vi "Main.vi"() -> ()   [LabVIEW 2024]
doc: "This template is for the Queued Message Handler design pattern.\n\nThe Event Handling Loop generates messages based on user interface actions.\n\nThe Message Handling Loop processes messages generated by the Event Handling Loop, or by other messages. The messages are string values, so new messages can be added easily to the Message Cases case structure in the Message Handling Loop. Each message cluster can also provide an optional value for Message Data, which is a variant that can be converted to whatever message-specific data is required."
uses:
  Torsjonsrigg/support/MotorBoolControlsIndicators.ctl
  Torsjonsrigg/support/MotorStatusIndicators.ctl
  Torsjonsrigg/controls/UI Data.ctl
  Torsjonsrigg/support/MotorSpeedControls.ctl
  Torsjonsrigg/support/MotorBoolControls.ctl
  <vilib>/Modbus/master/Create Master Instance (TCP).vi
  Torsjonsrigg/support/Message Queue/Enqueue Message (Single).vi
  <vilib>/Utility/error.llb/Error Cluster From Error Code.vi
  <vilib>/addons/control/pid/pid.llb/PID (DBL).vi
  <vilib>/ErrorRing/Error Ring.xnode
  <vilib>/Modbus/master/Modbus Master.lvclass
  Torsjonsrigg/support/Message Queue/Message Queue.lvlib
  Torsjonsrigg/support/User Event - Stop/User Event - Stop.lvlib
  <vilib>/addons/control/pid/NI_PID_pid.lvlib
panel:
  out "Mode Set":string
  in  "Index":i32
  out "Waveform 2":cluster{"X":dbl[], "Y":dbl[]}[](graph) caption="Waveform"
  in  "IP Address of PLC":string="192.168.1.36"
  in  "IPAddress of QuantumX":string="192.168.1.60"
  out "Setpoint Speed 2":dbl format="%.2f"
  out "?":cluster{"X":dbl[], "Y":dbl[]}[](graph)
  out "?":cluster{"X":dbl[], "Y":dbl[]}[](graph)
  out "Torque 1":dbl
  out "Speed Motor 2":dbl format="%.2f"
  out "Speed Motor1":dbl format="%.2f"
  out "Waveform":cluster{"X":dbl[], "Y":dbl[]}[](graph)
  out "Motor Status Indicators":T1
  out "Motor Bool Control Indicators":T2
  in  "Stop":bool
  in  "Setpoint Torque":dbl
  in  "Mode":string(combo)="Synchronus"
  in  "Setpoint Speed":dbl
  in  "Reset":bool
  in  "Start":bool
  in  "Exit":bool
  out "Status":string
  # "Torsion rig Control & Monitoring"
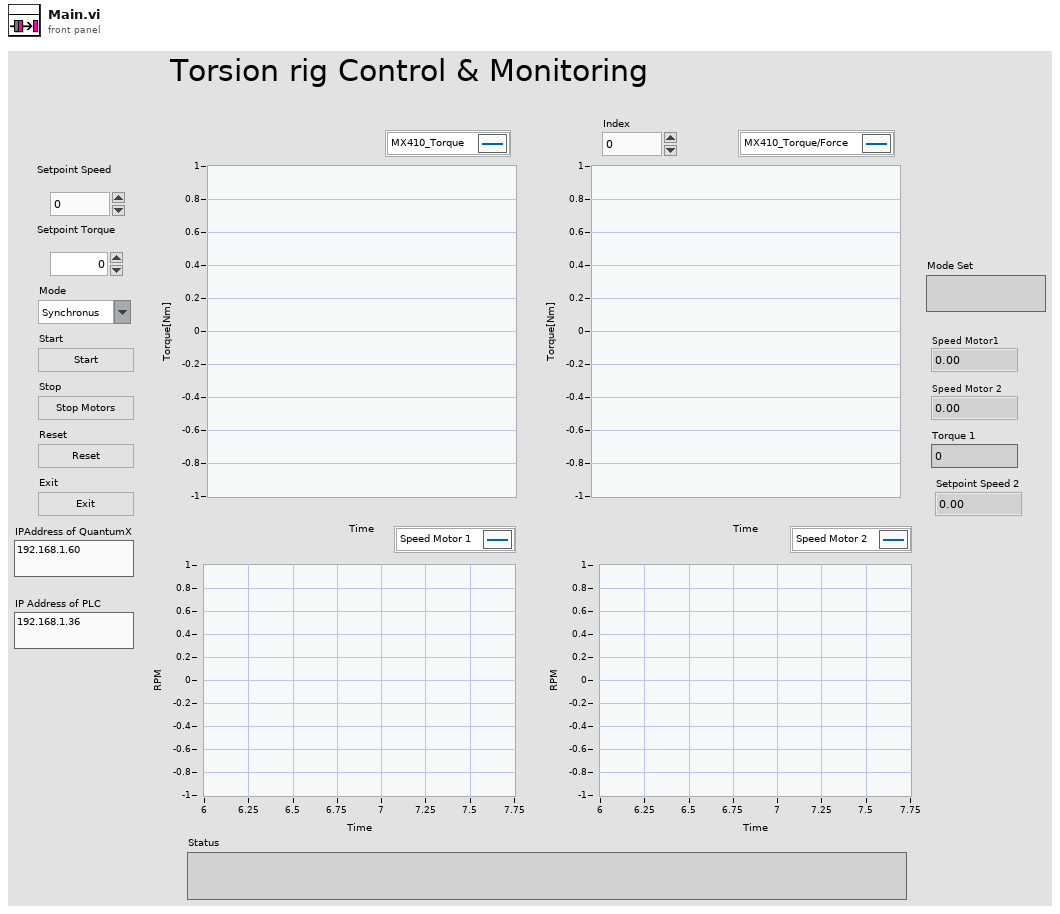
[diagram p1: front panel]
types:
  T1 = typedef "MotorStatusIndicators.ctl" = cluster{"Motor 1 Ok":bool, "Motor 2 ok":bool}
  T2 = typedef "MotorBoolControlsIndicators.ctl" = cluster{"Motors On":bool, "Reset":bool, "Motors Off":bool, "Start Motor 1 ":bool, "Start Motor 2":bool}
  T3 = typedef "MotorBoolControls.ctl" = cluster{"MotorsOn":bool, "Reset":bool, "MotorsOff":bool, "StartMotor1":bool, "StartMotor2":bool}
  T4 = typedef "MotorSpeedControls.ctl" = cluster{"SetSpeed1":dbl, "SetSpeed 2":dbl}
  T5 = typedef "UI Data.ctl" = cluster{"Boolean":bool, "Status":string, "Speed":u32, "Start Ref":refnum<vi>, "Reset":refnum<vi>, "Data Display Ref":refnum<vi>, "Exit Button Ref":refnum<vi>, "Torque":u32, "Async Ref":refnum<vi>, "Sync Ref":string}
  T6 = cluster{"Devices":refnum<k24>[], "Signals":refnum<k24>[]}
  T7 = typedef "Message Queue.lvlib/All Message Queues.ctl" = cluster{"UI":refnum<queue>, "Motor Controller":refnum<queue>, "Logging":refnum<queue>}
  T8 = enum8{"Enabled", "Disabled", "Disabled and Grayed Out"}
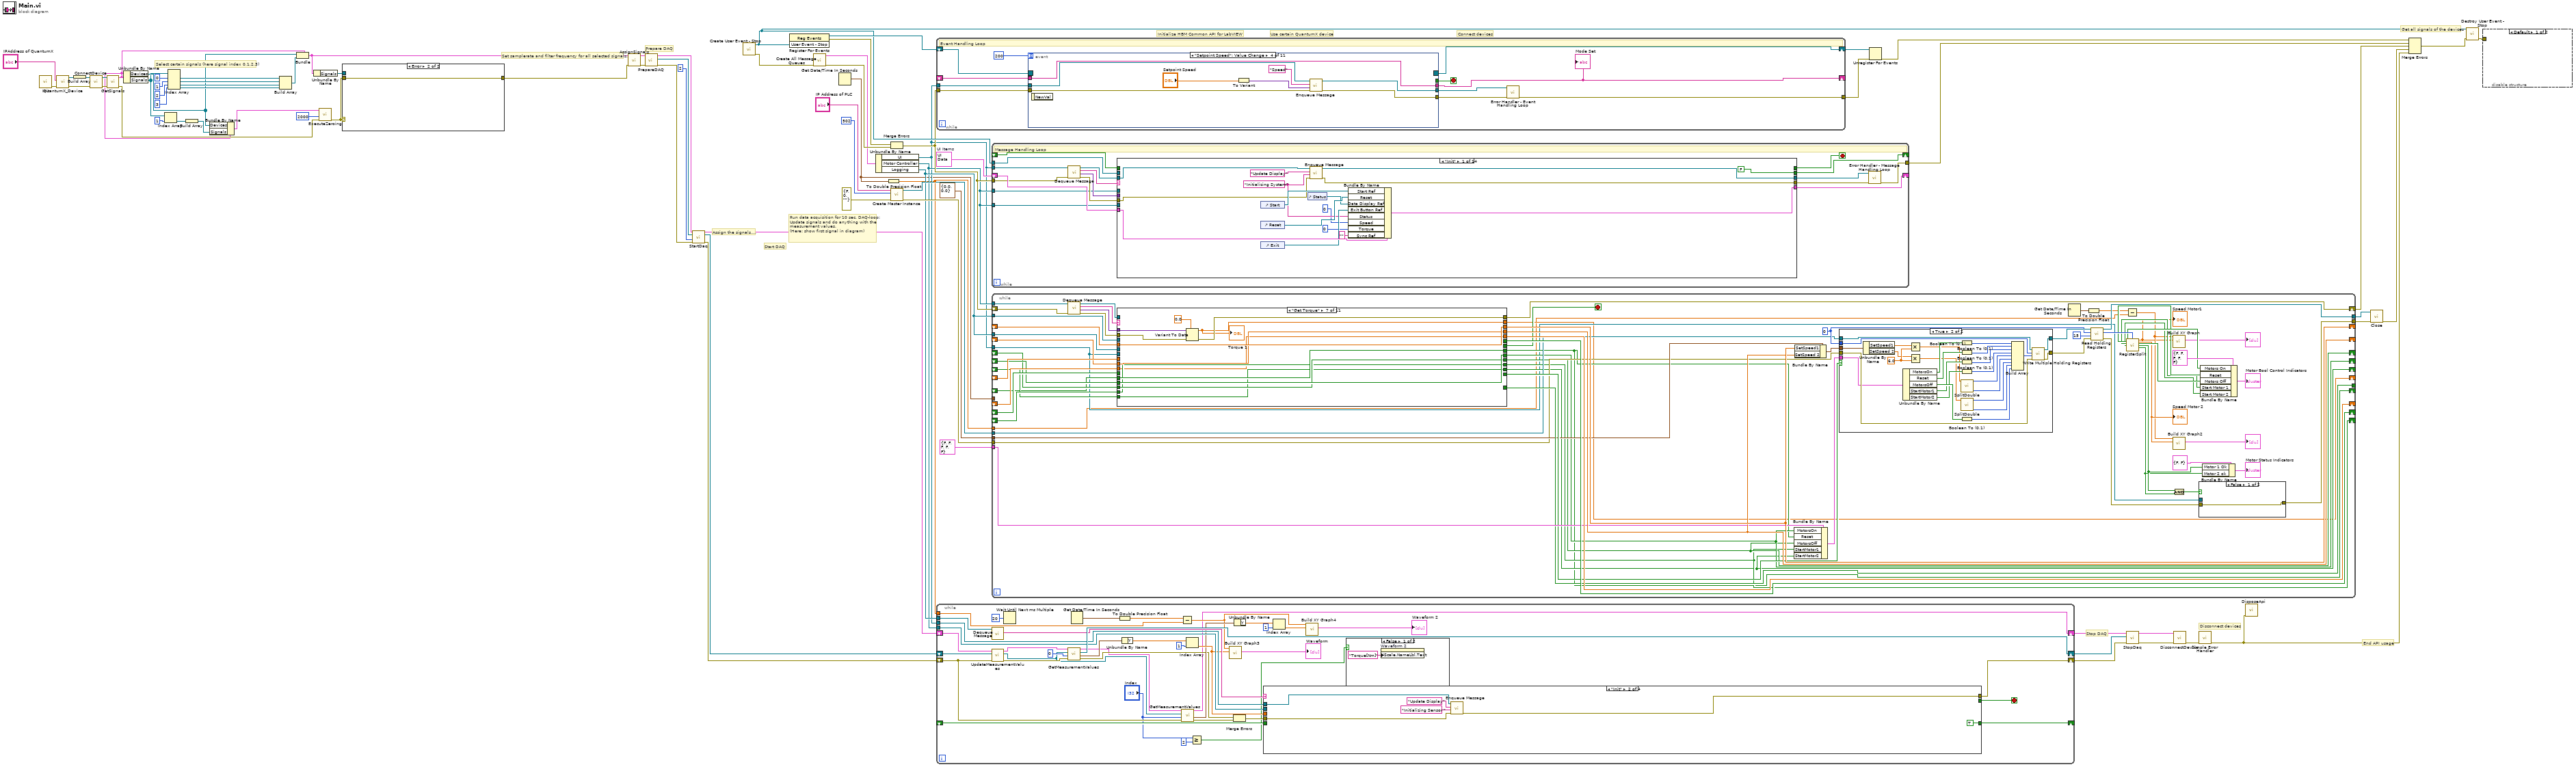
[diagram p0: block diagram]
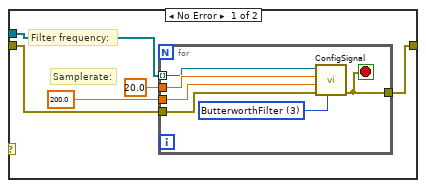
[diagram p2: hidden frame]
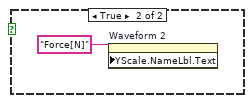
[diagram p3: hidden frame]
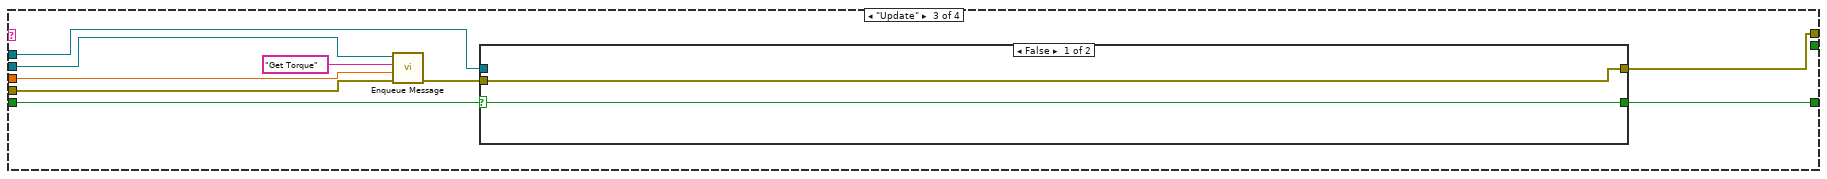
[diagram p5: hidden frame]
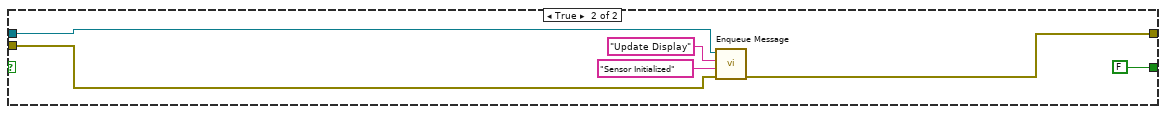
[diagram p6: hidden frame]
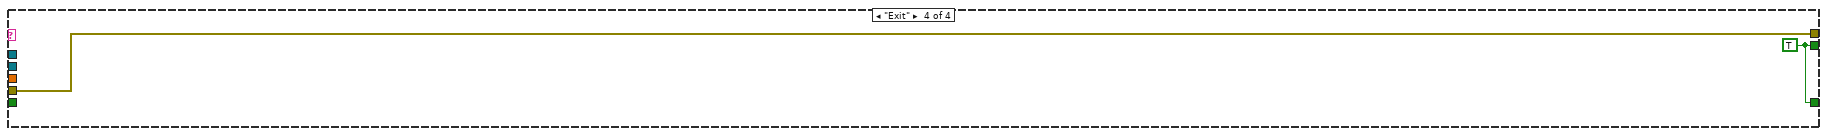
[diagram p7: hidden frame]
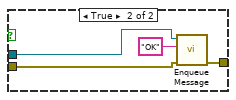
[diagram p8: hidden frame]
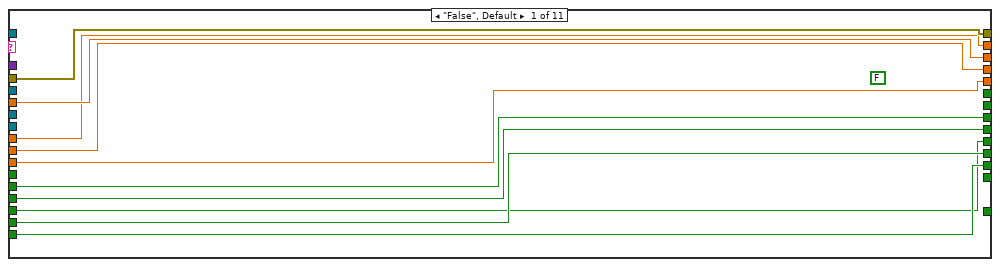
[diagram p10: hidden frame]
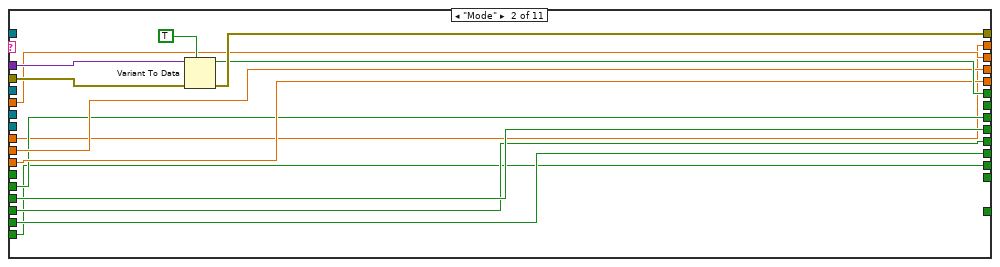
[diagram p11: hidden frame]
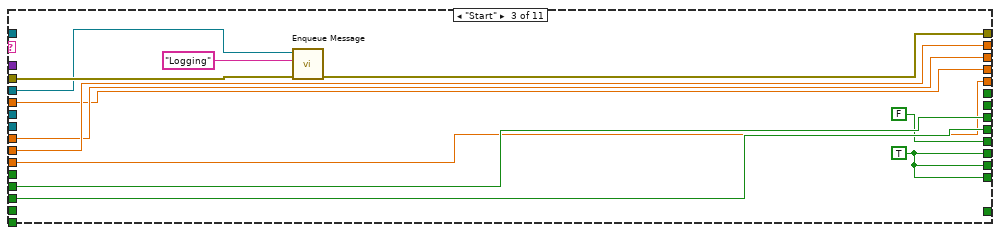
[diagram p12: hidden frame]
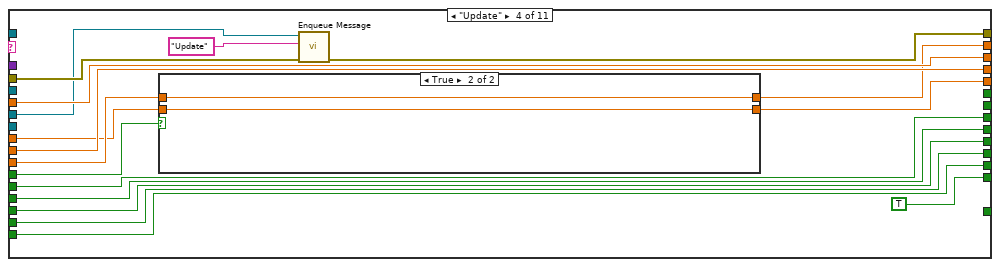
[diagram p13: hidden frame]
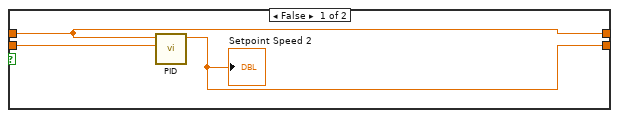
[diagram p14: hidden frame]
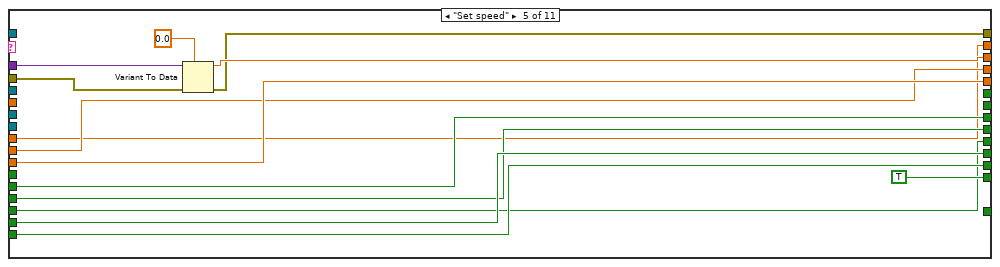
[diagram p15: hidden frame]
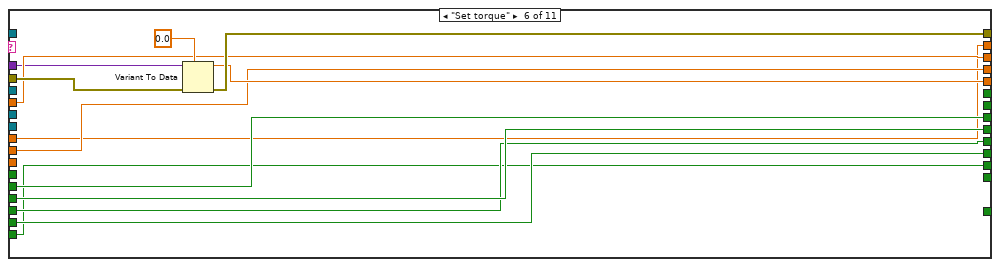
[diagram p16: hidden frame]
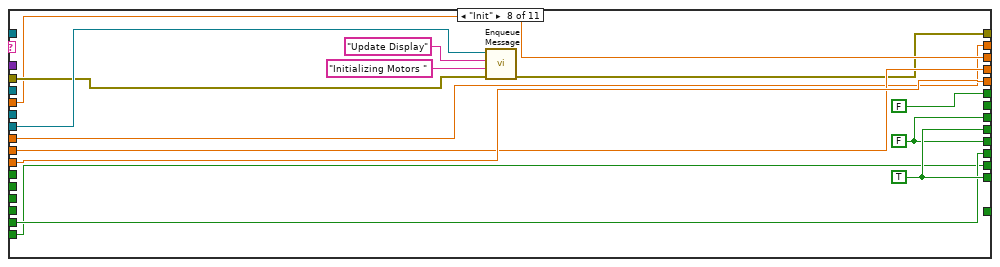
[diagram p17: hidden frame]
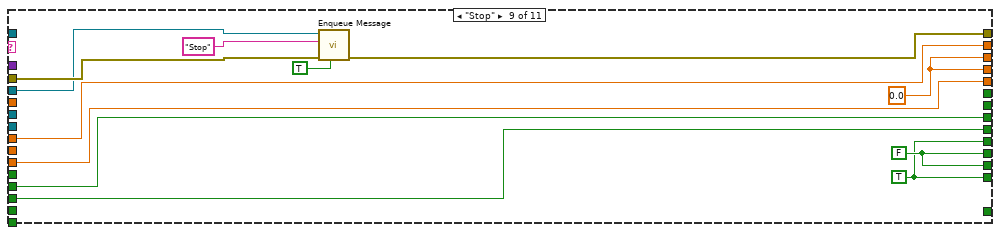
[diagram p18: hidden frame]
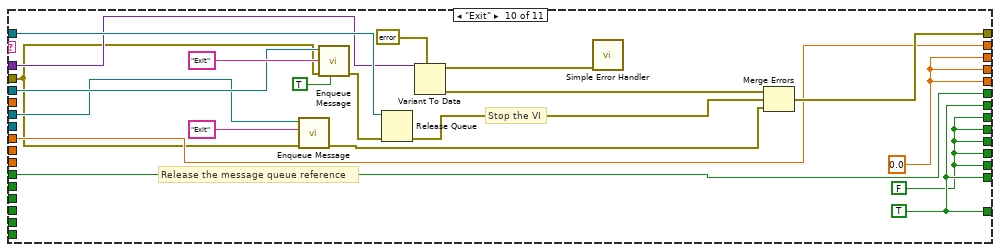
[diagram p19: hidden frame]
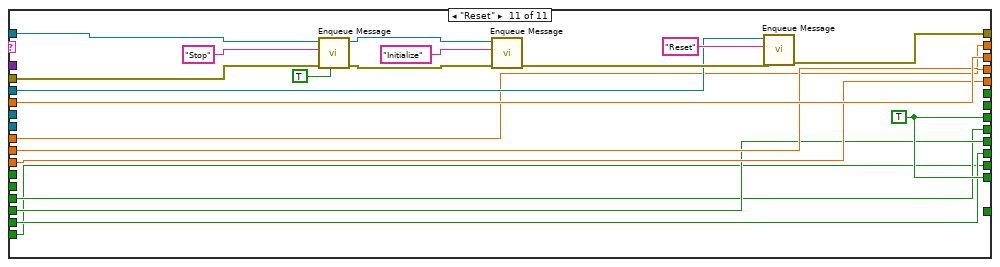
[diagram p20: hidden frame]
diagram:
  w70 = T5 {"Boolean"=FALSE, "Status"="", "Speed"=0, "Start Ref"=refnum, "Reset"=refnum, "Data Display Ref"=refnum, "Exit Button Ref"=refnum, "Torque"=0, "Async Ref"=refnum, "Sync Ref"=""}  # UI Items
  # "Set samplerate and filter frequency for all selected signals."
  # "Run data acquisition for 10 sec. DAQ-loop: Update signals and do anything with the  measurement values.\n(Here: show first signal in diagram)"
  # "Start DAQ"
  # "Prepare DAQ"
  # "Select certain signals (here signal index 0,1,2,3)"
  # "Assign the signals...."
  # "Disconnect devices"
  # "End API usage"
  # "Stop DAQ"
  # "Initialize HBM Common API for LabVIEW"
  # "Get all signals of the devices"
  # "Connect devices"
  # "Use certain QuantumX device"
  n1 = call <userlib>:"Init.vi"() -> ("Error out"=w22:errorcluster)  [unwired: 8 in, 2 out]
  n2 = call <userlib>:"QuantumX_Device.vi"("Error in"=w22, "IPAddress"="IPAddress of QuantumX") -> ("Error out"=w23:errorcluster, "Device"=w20:refnum<k24>)  [unwired: 6 in]
  n3 = Build Array(w20) -> (w19:refnum<k24>[])
  n4 = call <userlib>:"ConnectDevice.vi"("Error in"=w23, "Devices"=w19) -> ("Error out"=w36:errorcluster, "Devices"=w35:refnum<k24>[])  [unwired: 7 in, 1 out]
  n5 = call <userlib>:"GetSignals.vi"("Error in"=w36, "Devices"=w35) -> ("Error out"=w9:errorcluster, "DevicesAndSignals"=w7:T6)  [unwired: 8 in]
  n6 = Unbundle By Name(w7) -> ("Devices"=w11:refnum<k24>[], "Signals"=w10:refnum<k24>[])
  n7 = Index Array(array=w10, index=1) -> (element=w14:refnum<k24>)
  n8 = Index Array(array=w10, index #1=0 ("Index"), index #2=1 ("Index"), index #3=2 ("Index"), index #4=3 ("Index")) -> (element #1=w32:refnum<k24>, element #2=w31:refnum<k24>, element #3=w25:refnum<k24>, element #4=w24:refnum<k24>)
  n9 = Build Array(w14) -> (w15:refnum<k24>[])
  n10 = Bundle By Name(cluster=w7, "Devices"=w11, "Signals"=w15) -> (w6:T6)
  n11 = Build Array(w32, w31, w25, w24) -> (w30:refnum<k24>[])
  n12 = Bundle(cluster=w7, "Devices"=w11, "Signals"=w30) -> (w34:T6)
  n13 = Unbundle By Name(w34) -> ("Signals"=w43:refnum<k24>[])
  n14 = call <userlib>:"ExecuteZeroing.vi"("Error in"=w9, "NumberOfMeasurementValuesToUse"=2000, "DevicesAndSignals"=w6) -> ("Error out"=w8:errorcluster)  [unwired: 7 in, 1 out]
  n15 = case shown="Error" w8 {
    tunnel: w8 -> [w80 w87]
    tunnel: w43 -> [w79 _]
    tunnel: [w78 w87] -> w42
    frame No Error {
      # "Filter frequency:"
      # "Samplerate:"
      n16 = for {
        tunnel: w80 -> [w86]
        tunnel: 200.0 ("SampleRate") -> [w85]
        tunnel: 20.0 ("FilterFrequency") -> [w84]
        tunnel: w79 -> [w83] mode=indexing
        tunnel: [w82] -> w78
        stop <- w82 stop-if-true
        w81 = 3 items=["PresentFilter", "AutoFilter", "BesselFilter", "ButterworthFilter", "HighpassFilter", "LinearPhaseFilter", "NoFilter"] ("FilterType")
        n17 = call <userlib>:"ConfigSignal.vi"("FilterType"=w81, "Error in"=w86, "SampleRate"=w85, "FilterFrequency"=w84, "Signal"=w83) -> ("Error out"=w82:errorcluster)  [unwired: 6 in]
      }
    }
    frame Error {
    }
  }
  n18 = call <userlib>:"AssignSignals.vi"("Error in"=w42, "DevicesAndSignals"=w34) -> ("Error out"=w40:errorcluster, "DevicesAndSignals"=w41:T6)  [unwired: 8 in]
  n19 = call <userlib>:"PrepareDAQ.vi"("Error in"=w40, "DevicesAndSignals"=w41) -> ("Error out"=w37:errorcluster, "DaqMeasurement"=w38:refnum<k24>, "DevicesAndSignals"=w39:T6)  [unwired: 7 in]
  n20 = call <userlib>:"StartDaq.vi"("DevicesAndSignals"=w39, "DaqMeasurement"=w38, "AcquisitionMode"=2, "Error in"=w37) -> ("DevicesAndSignals"=w18:T6, "DaqMeasurement"=w17:refnum<k24>, "Error out"=w16:errorcluster)  [unwired: 7 in, 2 out]
  n21 = call "Create User Event - Stop.vi"() -> ("error out"=w64:errorcluster, "User Event - Stop"=w66:refnum<user-event>)  [unwired: 10 in]
  n22 = register-events(w66) -> (reference out=w67:refnum<event-registration>, error out=w65:errorcluster)  [unwired: 2 in]
  n23 = call "Create All Message Queues.vi"("error in (no error)"=w64) -> ("error out"=w75:errorcluster, "Message Queues out"=w63:T7)  [unwired: 9 in]
  n24 = Get Date/Time In Seconds() -> (seconds since 1Jan1904=w2:timestamp)
  n25 = Unbundle By Name(w63) -> ("UI"=w3:refnum<queue>, "Motor Controller"=w4:refnum<queue>, "Logging"=w5:refnum<queue>)
  n26 = To Double Precision Float(number=w2) -> (double precision float=w1:dbl)
  n27 = Merge Errors(w65, w75) -> (w61:errorcluster)
  n28 = call-poly <vilib>:"Create Master Instance.vi"("error in (no error)"=errorcluster {"status"=FALSE, "code"=0, "source"=""}, "port (502)"=u16 502, "address"="IP Address of PLC") -> ("error out"=w54:errorcluster, "TCP master instance"=w55:refnum<class "Modbus Master.lvclass">)  [unwired: 7 in]
  n29 = while {
    tunnel: w3 -> [w98]
    shift-right: [w96] -> w71
    shift-left: w67 -> [w97]
    tunnel: [w92] -> w68
    tunnel: w61 -> [w91]
    shift-right: [w89] -> _
    shift-left: _ -> [w88]
    stop <- w94 stop-if-true
    # "Event Handling Loop"
    n30 = event shown="[3] \"Setpoint Speed\": Value Change" {
      selector: w97 -> [_ _ _ _ _ _ _ _ _ _ _]
      dyn-events: [_ _ _ _ _ _ _ _ _ _ _] -> w96
      timeout: 200 -> [_ _ _ _ _ _ _ _ _ _ _]
      tunnel: [_ _ _ _ _ _ _ _ "Exit" _ TRUE ("Discard?")] -> w94
      tunnel: w98 -> [w103 w110 w117 w125 w132 w139 w143 w149 w158 w166 w171]
      tunnel: [w100 w108 w114 w122 w129 w138 w142 w146 w157 w165 w168] -> w95
      tunnel: [w102 w109 w116 w124 w131 w137 w143 w148 w156 w164 w171] -> w93
      tunnel: w91 -> [_ w107 w113 w121 w127 w134 w142 w147 w153 w161 w168]
      tunnel: [w99 "Mode" w112 w118 w126 w133 w141 w144 w151 w160 w167] -> w89
      tunnel: w88 -> [w99 _ w112 w118 w126 w133 w141 w144 w151 w160 w167]
      event "Start": Value Change {
        n31 = event-data() -> ()  [unwired: 1 in, 1 out]
        n32 = call-poly "Enqueue Message.vi"("Message"="Start", "Message Queue"=w103) -> ("error out"=w100:errorcluster, "dup Message Queue"=w102:refnum<queue>)  [unwired: 8 in]
      }
      event "Mode": Value Change {
        n33 = event-data() -> ()  [unwired: 1 in, 1 out]
        n34 = property on="Mode" class="CmbBox"("DisabledEnum"=T8."Disabled and Grayed Out" ("Disabled")) -> ()  [unwired: 2 in, 2 out]
        n35 = call-poly "Enqueue Message.vi"("error in (no error)"=w107, "Message Data"="Mode", "Message"="Mode", "Message Queue"=w110) -> ("error out"=w108:errorcluster, "dup Message Queue"=w109:refnum<queue>)  [unwired: 6 in]
      }
      event "Reset": Value Change {
        n36 = event-data() -> ()  [unwired: 1 in, 1 out]
        n37 = call-poly "Enqueue Message.vi"("error in (no error)"=w113, "Message"="Reset", "Message Queue"=w117) -> ("error out"=w114:errorcluster, "dup Message Queue"=w116:refnum<queue>)  [unwired: 7 in]
        n38 = property on="Mode" class="CmbBox"("DisabledEnum"=T8."Enabled" ("Disabled")) -> ()  [unwired: 2 in, 2 out]
      }
      event "Setpoint Speed": Value Change {
        n39 = event-data() -> ()  [unwired: 1 in, 1 out]
        n40 = To Variant(anything="Setpoint Speed") -> (Variant=w119:variant)
        n41 = call-poly "Enqueue Message.vi"("error in (no error)"=w121, "Message Data"=w119, "Message"="Speed", "Message Queue"=w125) -> ("error out"=w122:errorcluster, "dup Message Queue"=w124:refnum<queue>)  [unwired: 6 in]
      }
      event "Setpoint Torque": Value Change {
        n42 = event-data() -> ()  [unwired: 1 in, 1 out]
        n43 = call-poly "Enqueue Message.vi"("error in (no error)"=w127, "Message Data"="Setpoint Torque", "Message"="Torque", "Message Queue"=w132) -> ("error out"=w129:errorcluster, "dup Message Queue"=w131:refnum<queue>)  [unwired: 6 in]
      }
      event Panel Close? {
        n44 = event-data() -> ()  [unwired: 1 in, 1 out]
        n45 = call-poly "Enqueue Message.vi"("Priority Message? (F)"=TRUE, "error in (no error)"=w134, "Message"="Confirm Quit", "Message Queue"=w139) -> ("error out"=w138:errorcluster, "dup Message Queue"=w137:refnum<queue>)  [unwired: 6 in]
        n46 = event-data("Discard?"=TRUE) -> ()  [unwired: 1 in, 1 out]
      }
      event Application Instance Close {
        n47 = event-data() -> ()  [unwired: 1 in, 1 out]
      }
      event Timeout {
        n48 = event-data() -> ()  [unwired: 1 in, 3 out]
        n49 = call-poly "Enqueue Message.vi"("error in (no error)"=w147, "Message"="Update", "Message Queue"=w149) -> ("error out"=w146:errorcluster, "dup Message Queue"=w148:refnum<queue>)  [unwired: 7 in]
      }
      event "Exit": Value Change {
        n50 = event-data() -> ()  [unwired: 1 in, 1 out]
        n51 = call-poly "Enqueue Message.vi"("Priority Message? (F)"=TRUE, "error in (no error)"=w153, "Message"="Exit", "Message Queue"=w158) -> ("error out"=w157:errorcluster, "dup Message Queue"=w156:refnum<queue>)  [unwired: 6 in]
        n52 = property on="Mode" class="CmbBox"("DisabledEnum"=T8."Enabled" ("Disabled")) -> ()  [unwired: 2 in, 2 out]
      }
      event "Stop": Value Change {
        n53 = event-data() -> ()  [unwired: 1 in, 1 out]
        n54 = call-poly "Enqueue Message.vi"("Priority Message? (F)"=TRUE, "error in (no error)"=w161, "Message"="Stop", "Message Queue"=w166) -> ("error out"=w165:errorcluster, "dup Message Queue"=w164:refnum<queue>)  [unwired: 6 in]
        n55 = property on="Mode" class="CmbBox"("DisabledEnum"=T8."Enabled" ("Disabled")) -> ()  [unwired: 2 in, 2 out]
      }
      event User Event {
        n56 = event-data() -> ()  [unwired: 1 in, 1 out]
        n57 = local write "Status"("\"Exit\" button pressed" ("VI Stopped")) -> ()
      }
    }
    "Mode Set" <- w89
    n58 = call "Error Handler - Event Handling Loop.vi"("error in (no error)"=w95, "Message Queue"=w93) -> ("dup error in"=w92:errorcluster)  [unwired: 8 in, 1 out]
  }
  n59 = while {
    shift-right: [w175] -> w45
    shift-left: w18 -> [w209]
    shift-right: [w207] -> w50
    shift-left: w17 -> [w208]
    shift-right: [w199] -> w44
    shift-left: w16 -> [w180]
    tunnel: w5 -> [w210]
    tunnel: w4 -> [w200]
    tunnel: w3 -> [w202]
    shift-right: [w198] -> _
    shift-left: _ -> [w197]
    tunnel: w1 -> [w193]
    stop <- w201 stop-if-true
    n60 = call "Dequeue Message.vi"("Message Queue"=w210) -> ("Message"=w203:string)  [unwired: 7 in, 3 out]
    n61 = call <userlib>:"UpdateMeasurementValues.vi"("Error in"=w180, "DaqMeasurement"=w208, "DevicesAndSignals"=w209) -> ("Error out"=w204:errorcluster, "DaqMeasurement"=w181:refnum<k24>, "DevicesAndSignals"=w188:T6)  [unwired: 6 in]
    n62 = Wait Until Next ms Multiple(millisecond multiple=u32 20 ("Vielfache von ms")) -> ()  [unwired: 1 out]
    n63 = call <userlib>:"GetMeasurementValues.vi"("Error in"=w204, "Index"=0 ("Signal index to display"), "DaqMeasurement"=w181, "DevicesAndSignals"=w188) -> ("Error out"=w179:errorcluster, "Waveform"=w196:waveform(dbl), "DaqMeasurement"=w207:refnum<k24>, "DevicesAndSignals"=w176:T6)  [unwired: 2 in, 2 out]
    n64 = Get Date/Time In Seconds() -> (seconds since 1Jan1904=w195:timestamp)
    n65 = To Double Precision Float(number=w195) -> (double precision float=w194:dbl)
    n66 = Unbundle By Name(w196) -> ("Y"=w192:dbl[])
    n67 = Subtract(x=w194, y=w193) -> (x-y=w183:dbl)
    n68 = call <userlib>:"GetMeasurementValues.vi"("Error in"=w180, "Index"="Index", "DaqMeasurement"=w181, "DevicesAndSignals"=w176) -> ("Error out"=w177:errorcluster, "Waveform"=w184:waveform(dbl), "DevicesAndSignals"=w175:T6)  [unwired: 2 in, 3 out]
    n69 = Index Array(array=w192, index=1) -> (element=w189:dbl)
    n70 = Greater Or Equal?(x="Index", y=2) -> (x >= y?=w172:bool)
    n71 = call "Build XY Graph3"("Y Input"=w189, "X Input"=w183) -> ("XY Graph"=→"Waveform":cluster{"X":dbl[], "Y":dbl[]}[])  [unwired: 8 in, 1 out]
    n72 = Merge Errors(w179, w177) -> (w178:errorcluster)
    n73 = Unbundle By Name(w184) -> ("Y"=w187:dbl[])
    n74 = case shown="\"Init\"" w203 {
      tunnel: w202 -> [_ w220 w222 _]
      tunnel: [_ _ _ w238] -> w201
      tunnel: w178 -> [w214 w217 w229 w239]
      tunnel: w200 -> [_ _ w227 _]
      tunnel: [w214 w216 w224 w239] -> w199
      tunnel: [w213 TRUE w223 w238] -> w198
      tunnel: w197 -> [w213 _ w226 _]
      tunnel: w189 -> [_ _ w221 _]
      frame "False", Default {
      }
      frame "Init" {
        n75 = call-poly "Enqueue Message.vi"("error in (no error)"=w217, "Message Data"="Initializing Sensor ", "Message"="Update Display", "Message Queue"=w220) -> ("error out"=w216:errorcluster)  [unwired: 6 in, 1 out]
      }
      frame "Update" {
        n76 = call-poly "Enqueue Message.vi"("error in (no error)"=w229, "Message Data"=w221, "Message"="Get Torque", "Message Queue"=w227) -> ("error out"=w225:errorcluster)  [unwired: 6 in, 1 out]
        n77 = case shown="False" w226 {
          selector: w226 -> [w230 _]
          tunnel: [w231 w235] -> w224
          tunnel: w225 -> [w231 w234]
          tunnel: [w230 FALSE] -> w223
          tunnel: w222 -> [_ w232]
          frame False {
          }
          frame True {
            n78 = call-poly "Enqueue Message.vi"("error in (no error)"=w234, "Message Data"="Sensor Initialized", "Message"="Update Display", "Message Queue"=w232) -> ("error out"=w235:errorcluster)  [unwired: 6 in, 1 out]
          }
        }
      }
      frame "Exit" {
        w238 = TRUE
      }
    }
    n79 = Index Array(array=w187, index=1) -> (element=w182:dbl)
    n80 = call "Build XY Graph4"("Y Input"=w182, "X Input"=w183) -> ("XY Graph"=→"Waveform 2":cluster{"X":dbl[], "Y":dbl[]}[])  [unwired: 8 in, 1 out]
    n81 = case shown="False" w172 {
      frame False {
        n82 = property on="Waveform 2" class="XYGraph (strict)"("YScale.NameLbl.Text"="Torque[Nm]" ("Y Scale.Name Label.Text")) -> ()  [unwired: 2 in, 2 out]
      }
      frame True {
        n83 = property on="Waveform 2" class="XYGraph (strict)"("YScale.NameLbl.Text"="Force[N]" ("Y Scale.Name Label.Text")) -> ()  [unwired: 2 in, 2 out]
      }
    }
  }
  n84 = while {
    shift-right: [w255] -> _
    shift-left: w70 -> [w256]
    tunnel: w66 -> [w250]
    tunnel: w61 -> [w253]
    tunnel: [w252] -> w74
    tunnel: w3 -> [w248]
    tunnel: w4 -> [w245]
    tunnel: w4 -> [w242]
    shift-right: [w241] -> _
    shift-left: _ -> [w240]
    stop <- w254 stop-if-true
    # "Message Handling Loop"
    n85 = call "Dequeue Message.vi"("error in (no error)"=w253, "Message Queue"=w248) -> ("error out"=w246:errorcluster, "Message Data"=w247:variant, "Message"=w249:string, "dup Message Queue"=w244:refnum<queue>)  [unwired: 6 in]
    n86 = case "Message Cases" shown="\"Init\"" w249 {
      selector: w249 -> [_ w275 _ _ _ _ _ _ _ _ _ _ _ w388]
      tunnel: [w272 w277 w282 _ w290 w304 w316 w327 w337 w351 w357 w367 w382 w389] -> w251
      tunnel: w256 -> [w271 w280 w286 w288 w293 w309 w321 w332 w343 w352 w356 w368 w385 w390]
      tunnel: [w270 w280 w286 w288 w293 w309 w321 w332 w343 w352 w356 w368 w385 w390] -> w255
      tunnel: [_ _ _ _ _ _ _ _ _ _ _ _ TRUE _] -> w254
      tunnel: w250 -> [_ _ _ _ _ _ _ _ _ _ _ _ w381 _]
      tunnel: w247 -> [_ w279 _ _ _ w302 w314 _ _ w347 w355 _ w376 _]
      tunnel: w246 -> [w260 w278 w284 _ w291 _ w313 _ w338 w346 w354 _ w371 _]
      tunnel: w245 -> [_ w276 w285 _ _ w303 w317 w328 w336 _ _ _ w372 _]
      tunnel: w244 -> [w261 w274 _ _ _ w301 w312 w324 w335 w345 _ w363 w377 w387]
      tunnel: [w259 w274 _ _ _ w300 w311 w323 w334 w345 _ w362 _ w387] -> w243
      tunnel: w242 -> [_ _ _ _ w292 _ _ _ _ _ _ _ _ _]
      tunnel: [FALSE w273 w281 TRUE w289 w299 w310 w322 w333 w344 w353 FALSE w369 w386] -> w241
      tunnel: w240 -> [_ w273 w281 _ w289 w299 w310 w322 w333 w344 w353 _ w369 w386]
      frame "Init" {
        w264 = "Initializing System" ("Initial Message")
        # "Initialize - All initialization work should take place in this message, since other loops can potentially enqueue messages that execute immediately after this one."
        n87 = control-ref of="Start"() -> (w269:refnum<vi>)
        n88 = control-ref of="Reset"() -> (w268:refnum<vi>)
        n89 = control-ref of="Exit"() -> (w266:refnum<vi>)
        n90 = control-ref of="Status"() -> (w267:refnum<vi>)
        n91 = call-poly "Enqueue Message.vi"("error in (no error)"=w260, "Message Data"=w264, "Message"="Update Display", "Message Queue"=w261) -> ("error out"=w272:errorcluster, "dup Message Queue"=w259:refnum<queue>)  [unwired: 6 in]
        n92 = Bundle By Name(cluster=w271, "Start Ref"=w269, "Reset"=w268, "Data Display Ref"=w267, "Exit Button Ref"=w266, "Status"=w264, "Speed"=u32 0, "Torque"=u32 0, "Sync Ref"="") -> (w270:T5)
      }
      frame "Mode" {
        # "Something - Replace this message with functionality for your own application."
        n93 = call-poly "Enqueue Message.vi"("error in (no error)"=w278, "Message Data"=w279, "Message"=w275, "Message Queue"=w276) -> ("error out"=w277:errorcluster)  [unwired: 6 in, 1 out]
      }
      frame "Reset" {
        n94 = call-poly "Enqueue Message.vi"("error in (no error)"=w284, "Message"="Reset", "Message Queue"=w285) -> ("error out"=w282:errorcluster)  [unwired: 7 in, 1 out]
      }
      frame "Ok" {
      }
      frame "Update" {
        n95 = case shown="False" w289 {
          tunnel: w292 -> [_ w297]
          tunnel: w291 -> [w294 w296]
          tunnel: [w294 w295] -> w290
          frame False {
          }
          frame True {
            n96 = call-poly "Enqueue Message.vi"("error in (no error)"=w296, "Message"="Update", "Message Queue"=w297) -> ("error out"=w295:errorcluster)  [unwired: 7 in, 1 out]
          }
        }
      }
      frame "Speed" {
        # "Send string to \"Update Display\" message"
        n97 = call-poly "Enqueue Message.vi"("Message Data"=w302, "Message"="Set speed", "Message Queue"=w303) -> ("error out"=w305:errorcluster)  [unwired: 7 in, 1 out]
        n98 = call-poly "Enqueue Message.vi"("error in (no error)"=w305, "Message Data"="Starting Motor control" ("\"Do Something\" button pressed"), "Message"="Update Display", "Message Queue"=w301) -> ("error out"=w304:errorcluster, "dup Message Queue"=w300:refnum<queue>)  [unwired: 6 in]
      }
      frame "Torque" {
        # "Something - Replace this message with functionality for your own application."
        n99 = call-poly "Enqueue Message.vi"("error in (no error)"=w313, "Message Data"=w314, "Message"="Set torque", "Message Queue"=w317) -> ("error out"=w315:errorcluster)  [unwired: 6 in, 1 out]
        n100 = call-poly "Enqueue Message.vi"("error in (no error)"=w315, "Message Data"="Torque Changed" ("\"Do Something\" button pressed"), "Message"="Update Display", "Message Queue"=w312) -> ("error out"=w316:errorcluster, "dup Message Queue"=w311:refnum<queue>)  [unwired: 6 in]
      }
      frame "Stop" {
        (unwired) FALSE
        # "Send string to \"Update Display\" message"
        # "Something - Replace this message with functionality for your own application."
        n101 = call-poly "Enqueue Message.vi"("Priority Message? (F)"=TRUE, "Message"="Stop", "Message Queue"=w328) -> ("error out"=w326:errorcluster)  [unwired: 7 in, 1 out]
        n102 = call-poly "Enqueue Message.vi"("error in (no error)"=w326, "Message Data"="Stopping Motors" ("\"Do Something\" button pressed"), "Message"="Update Display", "Message Queue"=w324) -> ("error out"=w327:errorcluster, "dup Message Queue"=w323:refnum<queue>)  [unwired: 6 in]
      }
      frame "Start" {
        # "Send string to \"Update Display\" message"
        # "Something - Replace this message with functionality for your own application."
        n103 = call-poly "Enqueue Message.vi"("error in (no error)"=w338, "Message Data"="Starting " ("\"Do Something\" button pressed"), "Message"="Update Display", "Message Queue"=w335) -> ("error out"=w339:errorcluster, "dup Message Queue"=w334:refnum<queue>)  [unwired: 6 in]
        n104 = call-poly "Enqueue Message.vi"("error in (no error)"=w339, "Message"="Start", "Message Queue"=w336) -> ("error out"=w337:errorcluster)  [unwired: 7 in, 1 out]
      }
      frame "Update Display" {
        n105 = Variant To Data(error in=w346, type="", Variant=w347) -> (data=→"Status":string, error out=w349:errorcluster)
        n106 = Merge Errors(w349) -> (w351:errorcluster)
      }
      frame "Error" {
        # "Error - Display an error dialog. This message is sent by the \"Error Handler\" VIs at the end of other loops in this application."
        n107 = Variant To Data(error in=w354, type=errorcluster {"status"=FALSE, "code"=0, "source"=""} ("error constant"), Variant=w355) -> (data=w359:errorcluster, error out=w358:errorcluster)
        n108 = call <vilib>:"Simple Error Handler.vi"("error in (no error)"=w359) -> ()  [unwired: 4 in, 5 out]
        n109 = Merge Errors(w358) -> (w357:errorcluster)
      }
      frame "Confirm Quit" {
        # "Confirm Quit - Message that can confirm whether or not the user wants to exit the application."
        n110 = call-poly "Enqueue Message.vi"("Priority Message? (F)"=TRUE, "Message"="Exit", "Message Queue"=w363) -> ("error out"=w366:errorcluster, "dup Message Queue"=w362:refnum<queue>)  [unwired: 7 in]
        n111 = Merge Errors(w366) -> (w367:errorcluster)
      }
      frame "Exit" {
        # "Stop the VI"
        # "Release the message queue reference"
        # "Exit - Exit the application."
        n112 = Variant To Data(type=errorcluster {"status"=FALSE, "code"=0, "source"=""} ("error constant"), Variant=w376) -> (data=w378:errorcluster, error out=w375:errorcluster)  [unwired: 1 in]
        n113 = call <vilib>:"Simple Error Handler.vi"("error in (no error)"=w378) -> ()  [unwired: 4 in, 5 out]
        n114 = call-poly "Enqueue Message.vi"("Priority Message? (F)"=TRUE, "error in (no error)"=w371, "Message"="Exit", "Message Queue"=w372) -> ("error out"=w370:errorcluster)  [unwired: 6 in, 1 out]
        n115 = Release Queue(queue=w377, error in (no error)=w370) -> (error out=w383:errorcluster)  [unwired: 1 in, 2 out]
        n116 = call "Fire User Event - Stop.vi"("User Event - Stop"=w381) -> ("error out"=w380:errorcluster)  [unwired: 10 in]
        n117 = Merge Errors(w380, w383, w375) -> (w382:errorcluster)
      }
      frame Default {
        (unwired) FALSE
        (unwired) FALSE ("Sensors Initialized")
        # "'Default' case only runs if there is a message that isn't defined in any of the other cases.  Output a programming error."
        n118 = xnode "Error Ring"("parameter 0"=w388) -> ("error out"=w389:errorcluster)
      }
    }
    n119 = call "Error Handler - Message Handling Loop.vi"("error in (no error)"=w251, "Message Queue"=w243) -> ("dup error in"=w252:errorcluster)  [unwired: 8 in, 1 out]
  }
  n120 = while {
    tunnel: w5 -> [w450]
    tunnel: w3 -> [w408]
    tunnel: w4 -> [w462]
    shift-right: [w464] -> w62
    shift-left: w61 -> [w451]
    shift-right: [w449] -> _
    shift-left: _ -> [w457]
    shift-right: [w456] -> _
    shift-left: _ -> [w455]
    shift-right: [w448] -> _
    shift-left: _ -> [w454]
    shift-right: [w453] -> _
    shift-left: _ -> [w452]
    tunnel: T4 {"SetSpeed1"=0.0, "SetSpeed 2"=0.0} ("M;otor Speed Controls") -> [w428]
    tunnel: T3 {"MotorsOn"=FALSE, "Reset"=FALSE, "MotorsOff"=FALSE, "StartMotor1"=FALSE, "StartMotor2"=FALSE} ("Motor Bool Control") -> [w447]
    tunnel: [w446] -> _
    tunnel: w55 -> [w429]
    tunnel: w54 -> [w427]
    tunnel: [w426] -> w53
    tunnel: [w409] -> w52
    shift-right: [w423] -> _
    shift-left: _ -> [w422]
    shift-right: [w420] -> _
    shift-left: _ -> [w421]
    shift-right: [w419] -> _
    shift-left: _ -> [w416]
    shift-right: [w418] -> _
    shift-left: _ -> [w415]
    shift-right: [w417] -> _
    shift-left: _ -> [w414]
    shift-right: [w407] -> _
    shift-left: _ -> [w463]
    tunnel: w5 -> [w406]
    tunnel: w1 -> [w404]
    tunnel: w2 -> [_]
    stop <- w445 stop-if-true
    w440 = u16 0 ("starting address")
    n121 = call "Dequeue Message.vi"("error in (no error)"=w451, "Message Queue"=w462) -> ("error out"=w460:errorcluster, "Message Data"=w458:variant, "Message"=w461:string, "dup Message Queue"=w459:refnum<queue>)  [unwired: 6 in]
    n122 = case shown="\"Get Torque\"" w461 {
      tunnel: w460 -> [w508 w520 w534 w543 w569 w582 w595 w607 w620 w624 w659]
      tunnel: [w508 w519 w531 w542 w568 w581 w594 w602 w619 w630 w661] -> w464
      tunnel: w408 -> [_ _ _ _ _ _ _ w608 _ _ _]
      tunnel: w458 -> [_ w521 _ _ w565 w577 w591 _ _ w634 _]
      tunnel: [_ w518 _ _ _ _ _ FALSE _ w641 _] -> w453
      tunnel: [w507 w516 w525 w550 w570 w580 w593 w606 w617 w642 w652] -> w449
      tunnel: w457 -> [w507 w516 w524 w550 _ w580 w593 w606 _ _ w652]
      tunnel: [w506 w517 w523 w538 w567 w579 w585 w605 w618 w642 w651] -> w456
      tunnel: w455 -> [w506 w517 w523 w537 w567 _ w585 w605 w618 _ w651]
      tunnel: w459 -> [_ _ _ _ _ _ _ _ _ w635 w660]
      tunnel: w452 -> [_ _ _ w539 _ _ _ _ _ w641 _]
      tunnel: [w505 w515 w524 w549 w566 w578 w592 w604 w617 w642 w650] -> w448
      tunnel: w454 -> [w505 w515 w526 w549 w566 w578 w592 w604 _ _ w650]
      tunnel: w463 -> [w499 w509 w525 w536 w557 w571 _ w597 w611 w627 w643]
      tunnel: w450 -> [_ _ w532 _ _ _ _ _ w616 w633 w649]
      tunnel: [_ _ w529 TRUE ("Write") TRUE ("Reset") _ _ w601 w612 w629 w648] -> w430
      tunnel: [_ _ _ _ _ _ _ _ _ w629 _] -> w446
      tunnel: [_ _ _ _ _ _ _ _ _ w629 _] -> w445
      tunnel: [w500 w514 w530 w548 w558 w576 w590 w601 w615 w628 w646] -> w423
      tunnel: w422 -> [w500 w514 w530 w548 w558 w576 w590 _ w615 _ w646]
      tunnel: [w501 w513 w528 w547 w559 w575 w589 w600 w613 w628 w648] -> w417
      tunnel: w421 -> [w502 w512 _ w546 w560 w574 w588 _ _ _ w647]
      tunnel: [w502 w512 FALSE w546 w560 w574 w588 w600 w612 w628 w647] -> w420
      tunnel: [w503 w511 w529 w545 w562 w573 w587 w599 w614 w628 w645] -> w419
      tunnel: [w504 w510 w529 w544 w561 w572 w586 w598 w614 w628 w644] -> w418
      tunnel: w416 -> [w503 w511 _ w545 w562 w573 w587 w599 _ _ w645]
      tunnel: w415 -> [w504 w510 _ w544 w561 w572 w586 w598 _ _ w644]
      tunnel: w414 -> [w501 w513 w528 w547 w559 w575 w589 _ w613 _ _]
      tunnel: [w499 w509 w526 w535 w557 w571 w584 w597 w611 w627 w643] -> w407
      tunnel: w406 -> [_ _ _ w541 _ _ _ _ _ w626 _]
      frame "False", Default {
        (unwired) FALSE
      }
      frame "Mode" {
        n123 = Variant To Data(error in=w520, type=TRUE, Variant=w521) -> (data=w518:bool, error out=w519:errorcluster)
      }
      frame "Start" {
        w529 = TRUE ("Write")
        n124 = call-poly "Enqueue Message.vi"("error in (no error)"=w534, "Message"="Logging", "Message Queue"=w532) -> ("error out"=w531:errorcluster)  [unwired: 7 in, 1 out]
      }
      frame "Update" {
        n125 = case shown="True" w539 {
          tunnel: [w554 w556] -> w538
          tunnel: w536 -> [w553 w556]
          tunnel: w537 -> [w552 w555]
          tunnel: [w552 w555] -> w535
          frame False {
            n126 = call-poly <vilib>:"PID.vi"("process variable"=w553, "setpoint"=w552) -> ("output"=w554:dbl)  [unwired: 8 in, 1 out]
            "Setpoint Speed 2" <- w554
          }
          frame True {
          }
        }
        n127 = call-poly "Enqueue Message.vi"("error in (no error)"=w543, "Message"="Update", "Message Queue"=w541) -> ("error out"=w542:errorcluster)  [unwired: 7 in, 1 out]
      }
      frame "Set speed" {
        n128 = Variant To Data(error in=w569, type=0.0 ("number"), Variant=w565) -> (data=w570:dbl, error out=w568:errorcluster)
      }
      frame "Set torque" {
        n129 = Variant To Data(error in=w582, type=0.0, Variant=w577) -> (data=w579:dbl, error out=w581:errorcluster)
      }
      frame "Get Torque" {
        n130 = Variant To Data(error in=w595, type=0.0, Variant=w591) -> (data=w584:dbl, error out=w594:errorcluster)
        "Torque 1" <- w584
      }
      frame "Init" {
        w600 = FALSE
        w601 = TRUE
        n131 = call-poly "Enqueue Message.vi"("error in (no error)"=w607, "Message Data"="Initializing Motors ", "Message"="Update Display", "Message Queue"=w608) -> ("error out"=w602:errorcluster)  [unwired: 6 in, 1 out]
      }
      frame "Stop" {
        w614 = FALSE
        w612 = TRUE
        w617 = 0.0
        n132 = call-poly "Enqueue Message.vi"("Priority Message? (F)"=TRUE, "error in (no error)"=w620, "Message"="Stop", "Message Queue"=w616) -> ("error out"=w619:errorcluster)  [unwired: 6 in, 1 out]
      }
      frame "Exit" {
        w628 = FALSE
        w642 = 0.0
        w629 = TRUE
        # "Stop the VI"
        # "Release the message queue reference"
        n133 = call-poly "Enqueue Message.vi"("error in (no error)"=w624, "Message"="Exit", "Message Queue"=w626) -> ("error out"=w625:errorcluster)  [unwired: 7 in, 1 out]
        n134 = call-poly "Enqueue Message.vi"("Priority Message? (F)"=TRUE, "error in (no error)"=w624, "Message"="Exit", "Message Queue"=w633) -> ("error out"=w636:errorcluster)  [unwired: 6 in, 1 out]
        n135 = Release Queue(queue=w635, error in (no error)=w636) -> (error out=w631:errorcluster)  [unwired: 1 in, 2 out]
        n136 = Variant To Data(type=errorcluster {"status"=FALSE, "code"=0, "source"=""} ("error constant"), Variant=w634) -> (data=w639:errorcluster, error out=w632:errorcluster)  [unwired: 1 in]
        n137 = call <vilib>:"Simple Error Handler.vi"("error in (no error)"=w639) -> ()  [unwired: 4 in, 5 out]
        n138 = Merge Errors(w632, w631, w625) -> (w630:errorcluster)
      }
      frame "Reset" {
        w648 = TRUE ("Reset")
        n139 = call-poly "Enqueue Message.vi"("Priority Message? (F)"=TRUE, "error in (no error)"=w659, "Message"="Stop", "Message Queue"=w660) -> ("error out"=w655:errorcluster, "dup Message Queue"=w656:refnum<queue>)  [unwired: 6 in]
        n140 = call-poly "Enqueue Message.vi"("error in (no error)"=w655, "Message"="Initialize", "Message Queue"=w656) -> ("error out"=w653:errorcluster)  [unwired: 7 in, 1 out]
        n141 = call-poly "Enqueue Message.vi"("error in (no error)"=w653, "Message"="Reset", "Message Queue"=w649) -> ("error out"=w661:errorcluster)  [unwired: 7 in, 1 out]
      }
    }
    n142 = Bundle By Name(cluster=w447, "MotorsOn"=w423, "Reset"=w417, "MotorsOff"=w420, "StartMotor1"=w419, "StartMotor2"=w418) -> (w425:T3)
    n143 = Bundle By Name(cluster=w428, "SetSpeed1"=w449, "SetSpeed 2"=w448) -> (w424:T4)
    n144 = case shown="True" w430 {
      tunnel: w429 -> [w471 w474]
      tunnel: [w471 w498] -> w442
      tunnel: [w470 w497] -> w441
      tunnel: w427 -> [w470 w496]
      tunnel: w440 -> [_ w495]
      tunnel: w425 -> [_ w473]
      tunnel: w424 -> [_ w472]
      frame False {
      }
      frame True {
        w485 = 6.0 ("y")
        n145 = Unbundle By Name(w472) -> ("SetSpeed1"=w484:dbl, "SetSpeed 2"=w483:dbl)
        n146 = Unbundle By Name(w473) -> ("MotorsOn"=w494:bool, "Reset"=w493:bool, "MotorsOff"=w492:bool, "StartMotor1"=w491:bool, "StartMotor2"=w490:bool)
        n147 = Multiply(x=w484, y=w485) -> (x*y=w487:dbl)
        n148 = Multiply(x=w483, y=w485) -> (x*y=w486:dbl)
        n149 = Boolean To (0,1)(Boolean=w494) -> (0, 1=w489:i16)
        n150 = Boolean To (0,1)(Boolean=w493) -> (0, 1=w488:i16)
        n151 = Boolean To (0,1)(Boolean=w491) -> (0, 1=w482:i16)
        n152 = Boolean To (0,1)(Boolean=w490) -> (0, 1=w481:i16)
        n153 = Boolean To (0,1)(Boolean=w492) -> (0, 1=w476:i16)
        n154 = call "SplitDouble.vi"("number"=w487) -> ("Low"=w479:i16, "High"=w480:i16)  [unwired: 9 in]
        n155 = call "SplitDouble.vi"("number"=w486) -> ("Low"=w477:i16, "High"=w478:i16)  [unwired: 9 in]
        n156 = Build Array(w489, w488, w482, w481, w480, w479, w478, w477, w476) -> (w475:i16[])
        n157 = call-dynamic "Write Multiple Holding Registers.vi"("error in (no error)"=w496, "holding register values"=w475, "starting address"=w495, "Modbus master in"=w474) -> ("error out"=w497:errorcluster, "Modbus master out"=w498:refnum<class "Modbus Master.lvclass">)  [unwired: 6 in]
      }
    }
    n158 = Get Date/Time In Seconds() -> (seconds since 1Jan1904=w405:timestamp)
    n159 = To Double Precision Float(number=w405) -> (double precision float=w403:dbl)
    n160 = call-dynamic "Read Holding Registers.vi"("error in (no error)"=w441, "number of holding registers"=u16 15, "starting address"=w440, "Modbus master in"=w442) -> ("error out"=w410:errorcluster, "register values"=w443:u16[], "Modbus master out"=w426:refnum<class "Modbus Master.lvclass">)  [unwired: 5 in]
    n161 = Subtract(x=w403, y=w404) -> (x-y=w400:dbl)
    n162 = call "RegisterSplit.vi"("register values"=w443) -> ("[0] Motor1On"=w436:bool, "[1]Motor2On"=w435:bool, "[2]StartMotor1"=w434:bool, "[3]StartMotor2"=w433:bool, "[7]ReadSpeed1"=w399:dbl, "[8] ReadSpeed2"=w402:dbl, "[6] MotorsOff"=w437:bool, "[9]Motor1Ok"=w412:bool, "[10]Motor2Ok"=w411:bool)  [unwired: 8 in, 2 out]
    "Speed Motor1" <- w399
    "Speed Motor 2" <- w402
    n163 = call "Build XY Graph"("Y Input"=w399, "X Input"=w400) -> ("XY Graph"=→"?":cluster{"X":dbl[], "Y":dbl[]}[])  [unwired: 8 in, 1 out]
    n164 = call "Build XY Graph2"("Y Input"=w402, "X Input"=w400) -> ("XY Graph"=→"?":cluster{"X":dbl[], "Y":dbl[]}[])  [unwired: 8 in, 1 out]
    n165 = And(x=w412, y=w411) -> (x .and. y?=w413:bool)
    n166 = case shown="False" w413 {
      tunnel: w410 -> [w465 w469]
      tunnel: [w465 w468] -> w409
      tunnel: w408 -> [_ w467]
      frame False {
      }
      frame True {
        n167 = call-poly "Enqueue Message.vi"("error in (no error)"=w469, "Message"="OK", "Message Queue"=w467) -> ("error out"=w468:errorcluster)  [unwired: 7 in, 1 out]
      }
    }
    n168 = Bundle By Name(cluster=T2 {"Motors On"=FALSE, "Reset"=FALSE, "Motors Off"=FALSE, "Start Motor 1 "=FALSE, "Start Motor 2"=FALSE} ("Motor Bool Control Indicators"), "Motors On"=w436, "Reset"=w435, "Motors Off"=w437, "Start Motor 1"=w434, "Start Motor 2"=w433) -> (→"Motor Bool Control Indicators":T2)
    n169 = Bundle By Name(cluster=T1 {"Motor 1 Ok"=FALSE, "Motor 2 ok"=FALSE} ("Motor Status Indicators"), "Motor 1 Ok"=w412, "Motor 2 ok"=w411) -> (→"Motor Status Indicators":T1)
  }
  n170 = Unregister For Events(event registration refnum=w71, error in=w68) -> (error out=w72:errorcluster)
  n171 = call <userlib>:"StopDaq.vi"("Error in"=w44, "DaqMeasurement"=w50, "DevicesAndSignals"=w45) -> ("Error out"=w49:errorcluster, "DevicesAndSignals"=w48:T6)  [unwired: 7 in]
  n172 = call <userlib>:"DisconnectDevice.vi"("Error in"=w49, "DevicesAndSignals"=w48) -> ("Error out"=w47:errorcluster)  [unwired: 9 in]
  n173 = call <vilib>:"Simple Error Handler.vi"("error in (no error)"=w47) -> ("error out"=w46:errorcluster)  [unwired: 4 in, 4 out]
  n174 = call <userlib>:"DisposeApi.vi"("Error in"=w46) -> ()  [unwired: 10 in, 1 out]
  n175 = call-dynamic "Close.vi"("error in (no error)"=w52, "Modbus master in"=w53) -> ("error out"=w51:errorcluster)  [unwired: 9 in]
  n176 = Merge Errors(w72, w74, w62, w51, w46) -> (w73:errorcluster)
  n177 = call "Destroy User Event - Stop.vi"("error in (no error)"=w73, "User Event - Stop"=w66) -> ("error out"=w69:errorcluster)  [unwired: 9 in]
  n178 = disable-structure shown="Default" {
    disable-tunnel: w69 -> [_ _]
    frame condition #0 (active) {
    }
    frame condition #1 {
      # "Call Quit LabVIEW if running as a built application."
      n179 = Quit LabVIEW() -> ()  [unwired: 1 in]
    }
  }
